vi "LJstreamUD build header string.vi"(11 "Channel Config":T1={"# Channels"=4, "+Ch"=["0", "1", "2", "3", "4", "5", "6", "7"], "-Ch (U3)"=["31", "31", "31", "31", "31", "31", "31", "31"], "Ranges (UE9)"=[0, 0, 0, 0, 0, 0, 0, 0], "Scaling Equation"=["y=v0", "y=v1", "y=v2", "y=v3", "y=v4", "y=v5", "y=v6", "y=v7"]} {"Ranges (UE9)" items=["LJ_rgBIP5V", "LJ_rgUNI5V", "LJ_rgUNI2P5V", "LJ_rgUNI1P25V", "LJ_rgUNIP625V"]}) -> (3 "Header String":string)   [LabVIEW 2021]
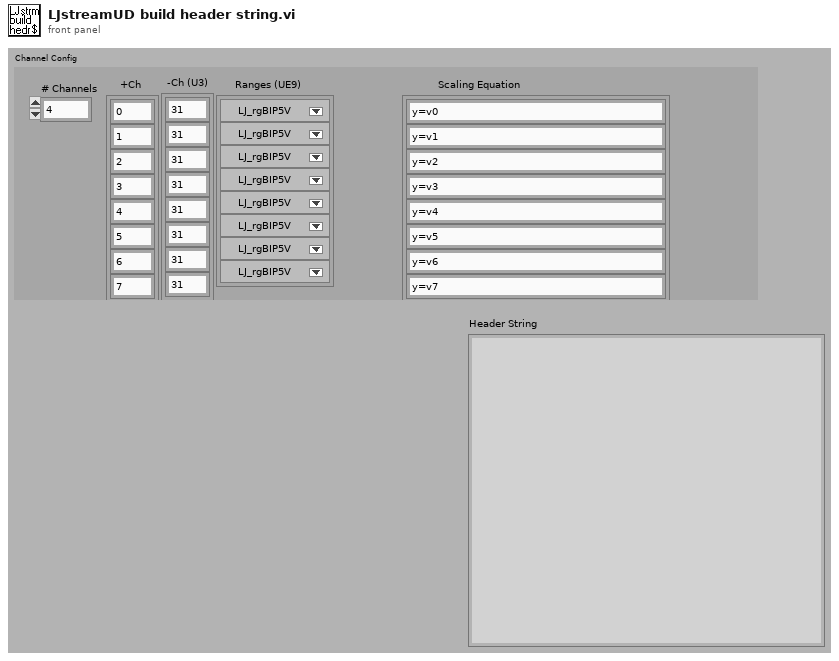
[diagram p1: front panel]
types:
  T1 = cluster{"# Channels":i32, "+Ch":string[], "-Ch (U3)":string[], "Ranges (UE9)":u16[], "Scaling Equation":string[]}
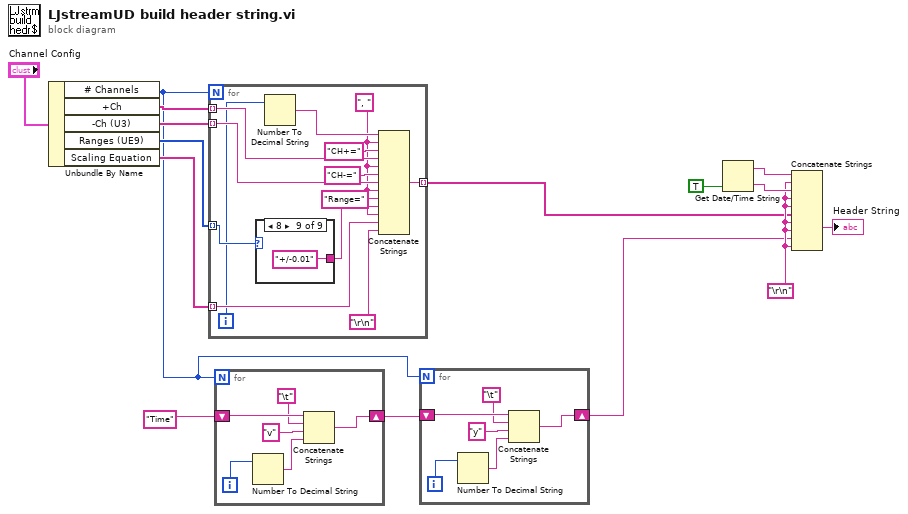
[diagram p0: block diagram]
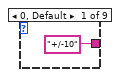
[diagram p2: hidden frame]
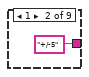
[diagram p3: hidden frame]
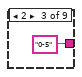
[diagram p4: hidden frame]
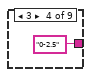
[diagram p5: hidden frame]
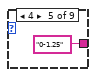
[diagram p6: hidden frame]
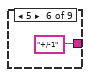
[diagram p7: hidden frame]
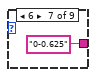
[diagram p8: hidden frame]
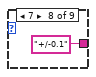
[diagram p9: hidden frame]
diagram:
  w13 = "\r\n"
  n1 = Unbundle By Name("Channel Config") -> ("# Channels"=w5:i32, "+Ch"=w10:string[], "-Ch (U3)"=w9:string[], "Ranges (UE9)"=w7:u16[], "Scaling Equation"=w8:string[])
  n2 = for {
    N: w5 -> [_]
    tunnel: w10 -> [w26] mode=indexing
    tunnel: w9 -> [w24] mode=indexing
    tunnel: w8 -> [w22] mode=indexing
    tunnel: w7 -> [w21] mode=indexing
    tunnel: [w17] -> w3 mode=indexing
    i -> [w16]
    w23 = ", " ("Substring")
    n3 = case shown="8" w21 {
      tunnel: ["+/-10" "+/-5" "0-5" "0-2.5" "0-1.25" "+/-1" "0-0.625" "+/-0.1" "+/-0.01"] -> w19
      frame 0, Default {
      }
      frame 1 {
      }
      frame 2 {
      }
      frame 3 {
      }
      frame 4 {
      }
      frame 5 {
      }
      frame 6 {
      }
      frame 7 {
      }
      frame 8 {
      }
    }
    n4 = Number To Decimal String(number=w16) -> (decimal integer string=w28:string)  [unwired: 1 in]
    n5 = Concatenate Strings(w28, w23, "CH+=" ("Substring"), w26, w23, "CH-=" ("Substring"), w24, w23, "Range=" ("Substring"), w19, w23, w22, "\r\n") -> (w17:string)
  }
  n6 = for {
    N: w5 -> [_]
    shift-right: [w42] -> w4
    shift-left: "Time" ("Substring") -> [w43]
    i -> [w39]
    n7 = Number To Decimal String(number=w39) -> (decimal integer string=w38:string)  [unwired: 1 in]
    n8 = Concatenate Strings(w43, "\t", "v" ("Substring"), w38) -> (w42:string)
  }
  n9 = for {
    N: w5 -> [_]
    shift-right: [w48] -> w2
    shift-left: w4 -> [w49]
    i -> [w45]
    n10 = Number To Decimal String(number=w45) -> (decimal integer string=w44:string)  [unwired: 1 in]
    n11 = Concatenate Strings(w49, "\t", "y" ("Substring"), w44) -> (w48:string)
  }
  n12 = Get Date/Time String(want seconds? (F)=TRUE) -> (date string=w15:string, time string=w14:string)  [unwired: 2 in]
  n13 = Concatenate Strings(w15, w13, w14, w13, w13, w3, w13, w13, w2, w13) -> (→"Header String":string)
